vi "Add Transfer with Children.vi"(4 "inline":bool, 5 "Transfer configuration":T1 {"channels"."string offset" format="%d bytes"}, 6 "Group Decimation (1)":u64, 7 "Transfer Group Status":refnum<class "Status.lvclass">, 8 "error in (no error)":errorcluster, 9 "Transfer":refnum<class "Transfer.lvclass">, 10 "parent tag":string, 11 "Application Data In":T6) -> (0 "error out":errorcluster, 3 "Application Data Out":T6)   [LabVIEW 2017, in "DSF Core.lvlib"]
uses:
  DSF Core.lvlib
  Main VI/Application Data.ctl
  <vilib>/NI/Memory Manager/Classes/Pointer/Pointer.lvclass
  Classes/Framework/Framework.lvclass
  Buffer Reader/Buffer Data.ctl
  Classes/Buffer/Buffer.lvclass
  C:/Program Files (x86)/National Instruments/LabVIEW 2017/vi.lib/NI/Memory Manager/Classes/Pointer/Pointer.lvclass
  Classes/Transfer Group Status/Status.lvclass
  Typedefs/DSF Engine Framework Configuration.ctl
  Typedefs/DSF Engine Plugin Configuration.ctl
  Typedefs/DSF Timing Info.ctl
  Typedefs/DSF Engine Plugin Thread Configuration.ctl
  Typedefs/DSF Settings Info.ctl
  Typedefs/DSF Engine Transfer Group Configuration.ctl
  Typedefs/DSF Direction.ctl
  Typedefs/DSF Engine Transfer Configuration.ctl
  Typedefs/DSF Byte Order.ctl
  Typedefs/DSF Engine Channel Configuration.ctl
  Typedefs/DSF Data Type.ctl
  Typedefs/DSF Timeout Behavior.ctl
  Classes/Transfer/Transfer.lvclass
  Classes/Transfer/Transfer.lvclass/Transfer.ctl
  Classes/Buffers/Buffers.lvclass/Buffers.ctl
  <vilib>/NI/Memory Manager/Classes/Pointer/Pointer.lvclass/Pointer.ctl
  ID to Tree Items/Tree Item Type.ctl
  Classes/Buffers/Get Inline Buffer.vi
  Classes/Buffers/Get Async Buffer.vi
  Add Buffer Channels.vi
  Classes/Buffer/Get Buffer Size.vi
  Sizeof.vi
  <vilib>/NI/Memory Manager/Classes/Pointer/Get Size.vi
  Classes/Buffer/Subset Buffer.vi
  Classes/Buffers/Buffers.lvclass
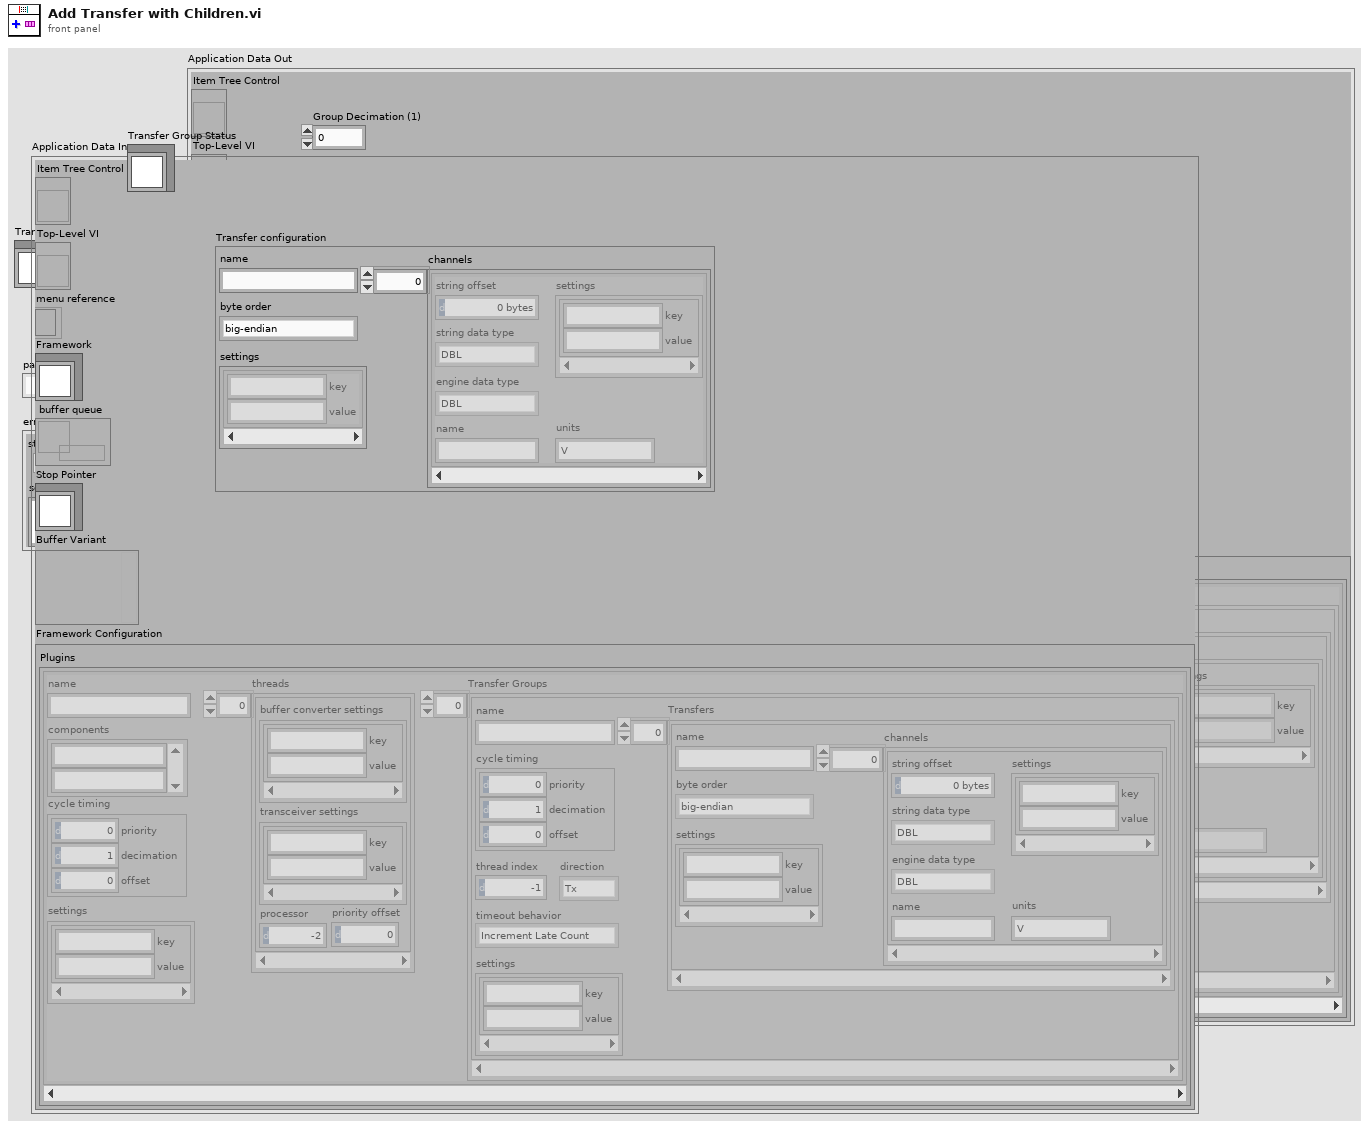
[diagram p1: front panel]
types:
  T1 = typedef "DSF Core.lvlib/DSF Engine Transfer Configuration.ctl" = cluster{"name":string, "byte order":T2, "settings":T3, "channels":T4[]}
  T2 = typedef "DSF Core.lvlib/DSF Byte Order.ctl" = enum8{"big-endian", "little-endian"}
  T3 = typedef "DSF Core.lvlib/DSF Settings Info.ctl" = cluster{"key":string, "value":string}[]
  T4 = typedef "DSF Core.lvlib/DSF Engine Channel Configuration.ctl" = cluster{"string offset":u64, "string data type":T5, "engine data type":T5, "name":string, "settings":T3, "units":string}
  T5 = typedef "DSF Core.lvlib/DSF Data Type.ctl" = enum8{"Bool", "SGL", "DBL", "I8", "I16", "I32", "I64", "U8", "U16", "U32", "U64"}
  T6 = typedef "DSF Core.lvlib/Application Data.ctl" = cluster{"Item Tree Control":refnum<vi>, "Top-Level VI":refnum<vi>, "menu reference":refnum<k9>, "Framework":refnum<class "Framework.lvclass">, "buffer queue":refnum<queue>, "Stop Pointer":refnum<class "Pointer.lvclass">, "Buffer Variant":variant, "Framework Configuration":T7}
  T7 = typedef "DSF Core.lvlib/DSF Engine Framework Configuration.ctl" = cluster{"Plugins":T8[]}
  T8 = typedef "DSF Core.lvlib/DSF Engine Plugin Configuration.ctl" = cluster{"name":string, "components":string[], "cycle timing":T9, "threads":T10[], "Transfer Groups":T11[], "settings":T3}
  T9 = typedef "DSF Core.lvlib/DSF Timing Info.ctl" = cluster{"priority":u64, "decimation":u64, "offset":u64}
  T10 = typedef "DSF Core.lvlib/DSF Engine Plugin Thread Configuration.ctl" = cluster{"buffer converter settings":T3, "transceiver settings":T3, "processor":i32, "priority offset":i16}
  T11 = typedef "DSF Core.lvlib/DSF Engine Transfer Group Configuration.ctl" = cluster{"name":string, "direction":T12, "cycle timing":T9, "thread index":i32, "settings":T3, "Transfers":T1[], "timeout behavior":T13}
  T12 = typedef "DSF Core.lvlib/DSF Direction.ctl" = enum8{"Tx", "Rx"}
  T13 = typedef "DSF Core.lvlib/DSF Timeout Behavior.ctl" = enum8{"Increment Late Count", "Throw Error"}
  T14 = typedef "DSF Core.lvlib/Buffer Data.ctl" = cluster{"Buffer":refnum<class "Buffer.lvclass">, "Status":refnum<class "Status.lvclass">, "decimation":u64, "avg bandwidth":dbl}
  T15 = typedef "DSF Core.lvlib/Tree Item Type.ctl" = enum16{"Framework", "Plugin Group", "Plugin", "Group", "Transfer", "Buffer", "Channel"}
  T16 = typedef "DSF Core.lvlib/Tree Item.ctl" = cluster{"Left Cell String":string, "Child Text":string[], "Child Tag":string, "Glyph Index":i32}
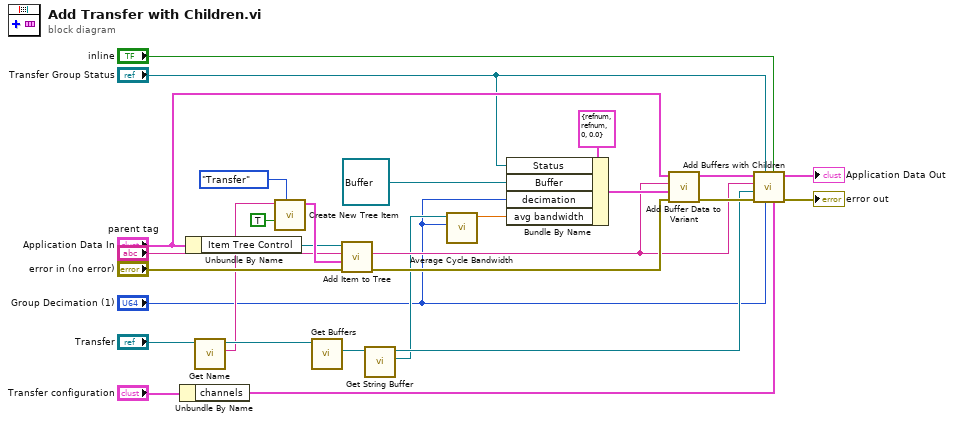
[diagram p0: block diagram]
diagram:
  n1 = Unbundle By Name("Transfer configuration") -> ("channels"=w2:T4[])
  n2 = Unbundle By Name("Application Data In") -> ("Item Tree Control"=w20:refnum<vi>)
  n3 = call "Get Name.vi"("Transfer in"="Transfer") -> ("name"=w21:string, "Transfer out"=w26:refnum<class "Transfer.lvclass">)  [unwired: 9 in]
  n4 = call "Create New Tree Item.vi"("Item Type"=Tree_Item_Type."Transfer", "found?"=TRUE, "Left Cell String"=w21) -> ("Item"=w28:T16)  [unwired: 7 in, 1 out]
  n5 = call "Get Buffers.vi"("Transfer in"=w26) -> ("Buffers"=w8:refnum<class "Buffers.lvclass">)  [unwired: 9 in, 1 out]
  n6 = call "Add Item to Tree.vi"("error in (no error)"="error in (no error)", "Item"=w28, "parent tag"="parent tag", "TreeControl in"=w20) -> ("error out"=w14:errorcluster, "new item tag"=w13:string)  [unwired: 5 in, 1 out]
  n7 = call "Get String Buffer.vi"("Buffers in"=w8) -> ("String Buffer"=w6:refnum<class "Buffer.lvclass">, "Buffers out"=w9:refnum<class "Buffers.lvclass">)  [unwired: 9 in]
  n8 = call "Average Cycle Bandwidth.vi"("Decimation"="Group Decimation (1)", "Buffer"=w6) -> ("avergage cycle bandwidth"=w7:dbl)  [unwired: 9 in]
  n9 = Bundle By Name(cluster=T14 {"Buffer"=refnum, "Status"=refnum, "decimation"=0, "avg bandwidth"=0.0} ("Buffer data"), "Status"="Transfer Group Status", "Buffer"=refnum<class "Buffer.lvclass"> refnum, "decimation"="Group Decimation (1)", "avg bandwidth"=w7) -> (w19:T14)
  n10 = call "Add Buffer Data to Variant.vi"("error in (no error)"=w14, "Buffer data"=w19, "tag"=w13, "Application Data In in"="Application Data In") -> ("error out"=w16:errorcluster, "Application Data In out"=w15:T6)  [unwired: 6 in]
  n11 = call "Add Buffers with Children.vi"("channels"=w2, "inline"="inline", "Decimation"="Group Decimation (1)", "Transfer Group Status"="Transfer Group Status", "error in (no error)"=w16, "Buffers"=w9, "parent tag"=w13, "Application Data In"=w15) -> ("error out"=→"error out":errorcluster, "Application Data out"=→"Application Data Out":T6)  [unwired: 2 in]
